vi "getStopMechanism.vi"(8 "error in (no error)":errorcluster, 11 "ExampleTask_StopNotifier in":refnum<class "ExampleTask_StopNotifier.lvclass">) -> (0 "error out":errorcluster, 2 "stopMechanism":refnum<class "ITaskStopMechanism.lvclass">, 3 "ExampleTask_StopNotifier out":refnum<class "ExampleTask_StopNotifier.lvclass">)   [LabVIEW 2023, in "ExampleTask_StopNotifier.lvclass"]
doc: "Returns the stop mechanism type used by the task."
uses:
  ExampleTask_StopNotifier.lvclass
  ExampleTask_StopNotifier.lvclass/ExampleTask_StopNotifier.ctl
  NotifierStopMechanism/NotifierStopMechanism.lvclass
  C:/projects/TLC_Daemon/source/NotifierStopMechanism/NotifierStopMechanism.lvclass
  C:/projects/TLC_Daemon/source/ITaskStopMechanism/ITaskStopMechanism.lvclass
  ITaskStopMechanism/ITaskStopMechanism.lvclass
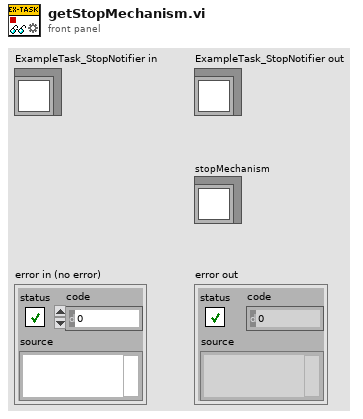
[diagram p1: front panel]
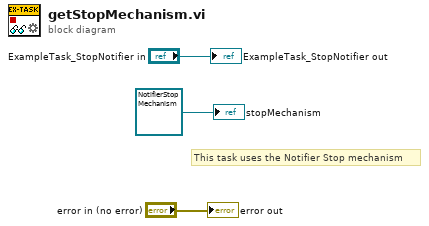
[diagram p0: block diagram]
diagram:
  # "This task uses the Notifier Stop mechanism"
  "error out" <- "error in (no error)"
  "ExampleTask_StopNotifier out" <- "ExampleTask_StopNotifier in"
  "stopMechanism" <- refnum<class "NotifierStopMechanism.lvclass"> refnum ("TLC_Daemon.lvlib:NotifierStopMechanism.lvclass")
